vi "read_msg_to_display.vi"(9 "pad_with_spaces (T)":bool=TRUE, 10 "separator (none)":T1(ring), 11 "Error in":refnum<class "Error.lvclass">) -> (2 "error_msg_to_display":string)   [LabVIEW 2023, in "Error Handling Interface.lvlib" / "Error.lvclass"]
doc: "Returns the <B>user-friendly</B> message to be used in displays or pop-ups"
uses:
  Error.lvclass
  Error.lvclass/Error.ctl
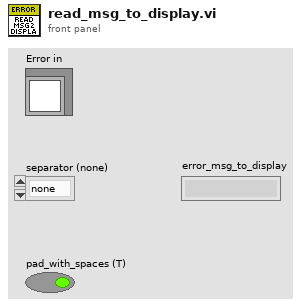
[diagram p1: front panel]
types:
  T1 = enum16{"none", "hifen", "fslash", "bslash", "vbar", "dot", "comma"}
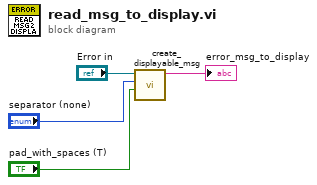
[diagram p0: block diagram]
diagram:
  n1 = call "create_displayable_msg.vi"("pad_with_spaces (T)"="pad_with_spaces (T)", "separator (none)"="separator (none)", "Error in"="Error in") -> ("error_msg_to_display"=→"error_msg_to_display":string)  [unwired: 8 in]
